vi "rpi_LabVIEW_RunControl.vi"() -> ()   [LabVIEW 2015]
uses:
  <vilib>/Rock Robotics/Network Tables/NT Read Boolean.vi
  <vilib>/Rock Robotics/Network Tables/NT Read Number.vi
  <vilib>/Rock Robotics/Network Tables/NT Write Boolean.vi
panel:
  out "RAM Total":dbl format="%#_6pBytes"
  out "Disk Total":dbl format="%#_6pBytes"
  out "Disk Free":dbl format="%#_6pBytes"
  out "Disk Usage":dbl format="%#_6pBytes"
  out "RAM Free":dbl format="%#_6pBytes"
  out "RAM Usage":dbl format="%#_6pBytes"
  out "Run Control":bool
  out "CPU Utilization":dbl(graph)
  out "RAM Usage":dbl(slide) scale=0.0..100.0
  out "Disk Usage":dbl(slide) scale=0.0..100.0
  out "CPU Utilization":dbl[](array[slide]) scale=0.0..100.0
  in  "Stop":bool
  in  "Shutdown":bool
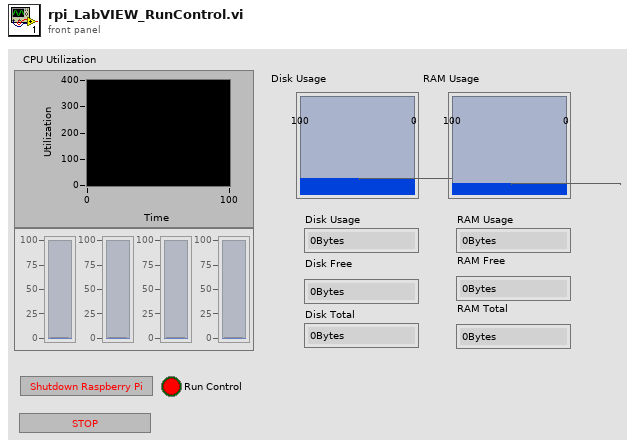
[diagram p1: front panel]
types:
  T1 = enum8{"Enabled", "Disabled", "Disabled and Grayed Out"}
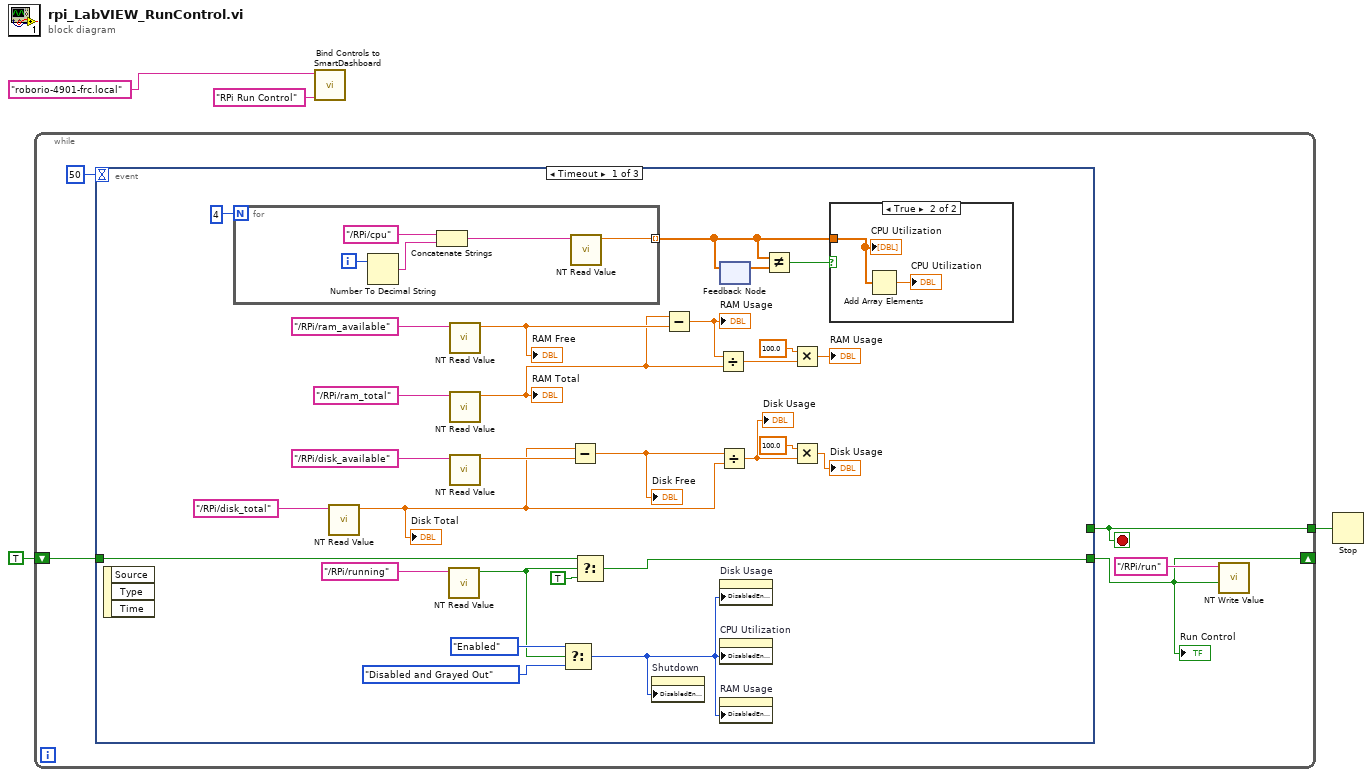
[diagram p0: block diagram]
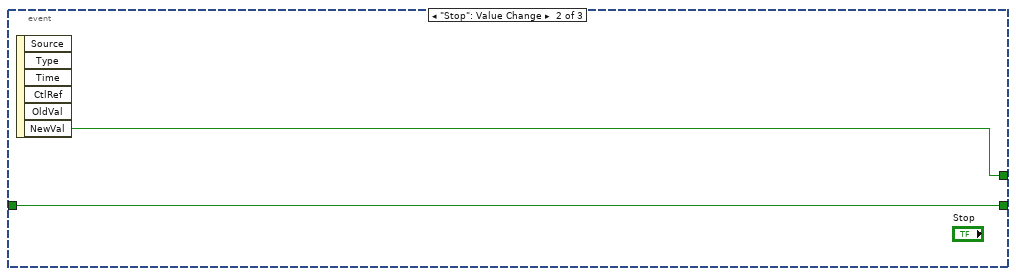
[diagram p3: hidden frame]
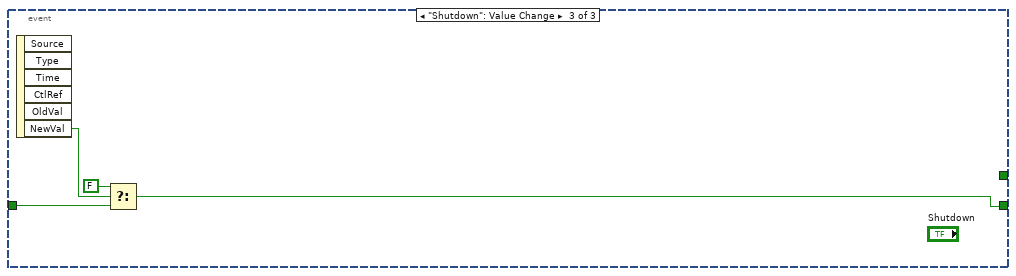
[diagram p4: hidden frame]
diagram:
  n1 = while {
    tunnel: [w9] -> w4
    shift-right: [w6] -> _
    shift-left: TRUE -> [w8]
    stop <- w9 stop-if-true
    n2 = event shown="[0] Timeout" {
      selector: _ -> [_ _ _]
      dyn-events: _ -> [_ _ _]
      timeout: 50 -> [_ _ _]
      tunnel: [_ w46 _] -> w9
      tunnel: w8 -> [w35 w45 w47]
      tunnel: [w31 w45 w48] -> w6
      event Timeout {
        n3 = event-data() -> ()  [unwired: 1 in, 3 out]
        n4 = for {
          N: 4 -> [_]
          tunnel: [w40] -> w15 mode=indexing
          i -> [w42]
          n5 = Number To Decimal String(number=w42) -> (decimal integer string=w41:string)  [unwired: 1 in]
          n6 = Concatenate Strings("/RPi/cpu" ("string"), w41) -> (w44:string)
          n7 = call-poly <vilib>:"NT Read Value.vi"("Name"=w44) -> ("Numeric"=w40:dbl)  [unwired: 9 in, 1 out]
        }
        n8 = call-poly <vilib>:"NT Read Value.vi"("Name"="/RPi/disk_total") -> ("Numeric"=w11:dbl)  [unwired: 9 in, 1 out]
        "Disk Total" <- w11
        n9 = call-poly <vilib>:"NT Read Value.vi"("Name"="/RPi/running") -> ("Boolean"=w32:bool)  [unwired: 9 in, 1 out]
        n10 = call-poly <vilib>:"NT Read Value.vi"("Name"="/RPi/ram_available") -> ("Numeric"=w19:dbl)  [unwired: 9 in, 1 out]
        "RAM Free" <- w19
        n11 = call-poly <vilib>:"NT Read Value.vi"("Name"="/RPi/ram_total") -> ("Numeric"=w10:dbl)  [unwired: 9 in, 1 out]
        "RAM Total" <- w10
        n12 = call-poly <vilib>:"NT Read Value.vi"("Name"="/RPi/disk_available") -> ("Numeric"=w20:dbl)  [unwired: 9 in, 1 out]
        n13 = Select(t=T1."Enabled" ("Disabled"), s=w32, f=T1."Disabled and Grayed Out" ("Disabled")) -> (s? t:f=w17:T1)
        n14 = Subtract(x=w11, y=w20) -> (x-y=w12:dbl)
        "Disk Free" <- w12
        n15 = Select(t=w35, s=w32, f=TRUE) -> (s? t:f=w31:bool)
        n16 = property on="Shutdown" class="Bool"("DisabledEnum"=w17) -> ()  [unwired: 2 in, 2 out]
        n17 = Subtract(x=w10, y=w19) -> (x-y=w18:dbl)
        "RAM Usage" <- w18
        n18 = Divide(x=w18, y=w10) -> (x/y=w25:dbl)
        n19 = Divide(x=w12, y=w11) -> (x/y=w13:dbl)
        "Disk Usage" <- w13
        n20 = feedback-in #1(w15) -> ()
        n21 = feedback #1() -> (w16:dbl[])  [unwired: 1 in]
        n22 = property on="Disk Usage" class="Slide (strict)"("DisabledEnum"=w17) -> ()  [unwired: 2 in, 2 out]
        n23 = property on="CPU Utilization" class="Arr (strict)"("DisabledEnum"=w17) -> ()  [unwired: 2 in, 2 out]
        n24 = property on="RAM Usage" class="Slide (strict)"("DisabledEnum"=w17) -> ()  [unwired: 2 in, 2 out]
        n25 = Not Equal?(x=w15, y=w16) -> (x != y?=w14:bool)
        n26 = Multiply(x=100.0, y=w25) -> (x*y=→"RAM Usage":dbl)
        n27 = Multiply(x=100.0, y=w13) -> (x*y=→"Disk Usage":dbl)
        n28 = case shown="True" w14 {
          tunnel: w15 -> [_ w39]
          frame False {
          }
          frame True {
            n29 = Add Array Elements(numeric array=w39) -> (sum=→"CPU Utilization":dbl)
            "CPU Utilization" <- w39
          }
        }
      }
      event "Stop": Value Change {
        n30 = event-data() -> ("NewVal"=w46:bool)  [unwired: 1 in, 5 out]
      }
      event "Shutdown": Value Change {
        n31 = event-data() -> ("NewVal"=w49:bool)  [unwired: 1 in, 5 out]
        n32 = Select(t=FALSE, s=w49, f=w47) -> (s? t:f=w48:bool)
      }
    }
    "Run Control" <- w6
    n33 = call-poly <vilib>:"NT Write Value.vi"("Boolean"=w6, "Name"="/RPi/run") -> ()  [unwired: 9 in, 1 out]
  }
  n34 = call <vilib>:"Bind Controls to SmartDashboard.vi"("Client Name"="RPi Run Control", "Server IP Address"="roborio-4901-frc.local") -> ()  [unwired: 10 in]
  n35 = Stop(stop? (T)=w4) -> ()
